vi "Project Save.vi"(8 "error in":errorcluster, 11 "File Path":path) -> (0 "error out":errorcluster caption="错误输出", 3 "selected path":path)   [LabVIEW 2016]
uses:
  DAQ-List/Controls/DAQListOperation.ctl
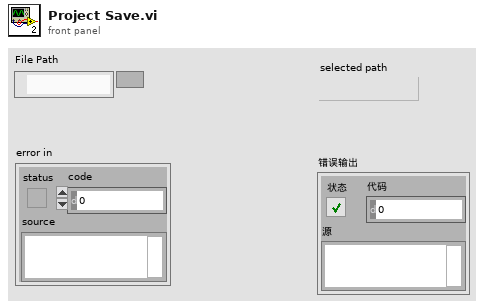
[diagram p1: front panel]
types:
  T1 = typedef "DAQListOperation.ctl" = enum16{"Init", "Clear", "Update Data", "Update CH Name", "Set List Property", "Get CHTag[]"}
  T2 = typedef "PSCHN_Card Para.ctl" = cluster{"Module Type":string, "Module Name":string, "ModuSN":string, "ModuIP":string, "Used?":bool, "Connected":bool, "Timing*":cluster{"Sample Rate":dbl}, "Channels":T3[]}
  T3 = typedef "PSCHN_Channel Para.ctl" = cluster{"CHTag*":string, "Used?*":bool, "CHName":string, "Unit":string, "斜率":dbl, "截距":dbl}
  T4 = typedef "Global para Config.ctl" = cluster{"连续存储设置":cluster{"Save Mode":i32, "Sel Save Mode":i32, "FolderPath":path, "Filename":string, "Explation":string, "AutoPoint":i32, "Template":path}, "Latest Prj":path, "Tdms Ref*":refnum<k34>, "默认波形图个数":u8, "列表列数":u8}
  T5 = typedef "PSVCH_VCH Info.ctl" = cluster{"Tag":string[], "Tag String":string[], "Name":string[], "Enable":bool[], "Formula":string[], "Unit":string[], "Save":bool[], "Time":i64[]}
  T6 = cluster{"DispXml[]":string[], "VCH Out":T5, "_Para":T4, "Cards":T2[], "CHTag[]":string[]}
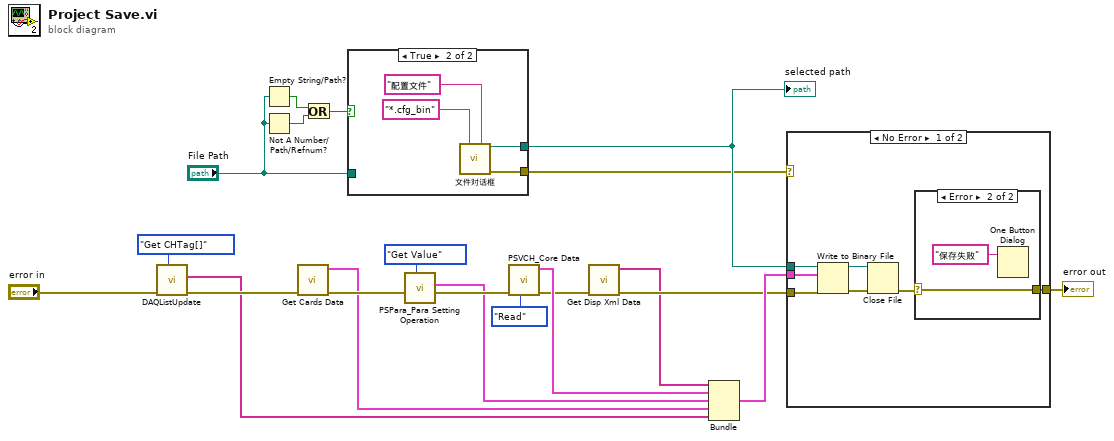
[diagram p0: block diagram]
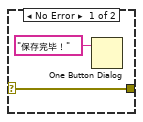
[diagram p2: hidden frame]
diagram:
  n1 = call "DAQListUpdate.vi"("Comm"=DAQListOperation."Get CHTag[]", "error in (no error)"="error in") -> ("error out"=w2:errorcluster, "CHTag[]"=w1:string[])  [unwired: 7 in, 1 out]
  n2 = Empty String/Path?(string/path="File Path") -> (empty?=w11:bool)
  n3 = Not A Number/Path/Refnum?(number/path/refnum="File Path") -> (NaN/Path/Refnum?=w10:bool)
  n4 = call "Get Cards Data.vi"("error in"=w2) -> ("error out"=w13:errorcluster, "Cards"=w5:T2[])  [unwired: 9 in]
  n5 = Or(x=w11, y=w10) -> (x .or. y?=w9:bool)
  n6 = case shown="True" w9 {
    tunnel: [w23 w25] -> w8
    tunnel: "File Path" -> [w23 _]
    tunnel: [_ w24] -> w6
    frame False {
    }
    frame True {
      n7 = call "文件对话框"("pattern (all files)"="*.cfg_bin", "pattern label"="配置文件") -> ("selected path"=w25:path, "error out"=w24:errorcluster)  [unwired: 10 in, 2 out]
    }
  }
  "selected path" <- w8
  n8 = call "PSPara_Para Setting Operation.vi"("Operation"=enum16{"Set Value", "Get Value", "Initialize"}."Get Value", "error in (no error)"=w13) -> ("error out"=w20:errorcluster, "_Para"=w17:T4)  [unwired: 8 in]
  n9 = call "PSVCH_Core Data.vi"("Oper"=enum16{"Init", "Read", "Write"}."Read", "Error In (no error)"=w20) -> ("Error Out"=w16:errorcluster, "VCH Out"=w18:T5)  [unwired: 8 in]
  n10 = call "Get Disp Xml Data.vi"("error in"=w16) -> ("error out"=w15:errorcluster, "DispXml[]"=w14:string[])  [unwired: 9 in]
  n11 = Bundle("DispXml[]"=w14, "VCH Out"=w18, "_Para"=w17, "Cards"=w5, "CHTag[]"=w1) -> (w19:T6)  [unwired: 1 in]
  n12 = case shown="No Error" w6 {
    tunnel: w19 -> [w34 _]
    tunnel: w15 -> [w31 w39]
    tunnel: [w30 w39] -> w12
    tunnel: w8 -> [w29 _]
    frame No Error {
      n13 = Write to Binary File(file (use dialog)=w29, data=w34, error in=w31) -> (refnum out=w32:refnum<file>, error out=w33:errorcluster)  [unwired: 3 in, 1 out]
      n14 = Close File(refnum=w32, error in=w33) -> (error out=w28:errorcluster)  [unwired: 1 out]
      n15 = case shown="Error" w28 {
        selector: w28 -> [w36 w38]
        tunnel: [w36 w38] -> w30
        frame No Error {
          n16 = One Button Dialog(message="保存完毕！" ("消息")) -> ()  [unwired: 1 in, 1 out]
        }
        frame Error {
          n17 = One Button Dialog(message="保存失败" ("消息")) -> ()  [unwired: 1 in, 1 out]
        }
      }
    }
    frame Error {
    }
  }
  "error out" <- w12
